vi "Drag-to-Dynamic.vi"(10 "Drag In":dbl, 11 "Waveform":waveform(dbl)) -> (3 "Dynamic Data Type":dynamicdata(waveform))   [LabVIEW 2025]
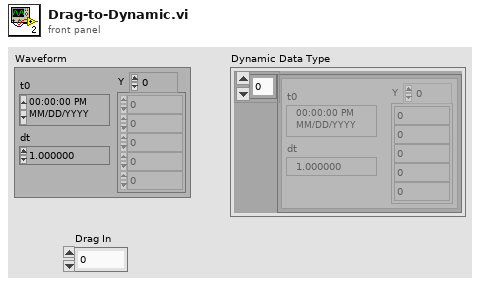
[diagram p1: front panel]
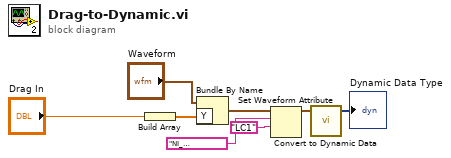
[diagram p0: block diagram]
diagram:
  n1 = Build Array("Drag In") -> (w8:dbl[])
  n2 = Bundle By Name(cluster="Waveform", "Y"=w8) -> (w2:waveform(dbl))
  n3 = Set Waveform Attribute(5:"LC1" ("name"), 6:"NI_ChannelName" ("name"), 7:w2) -> (3:w5:waveform(dbl))  [unwired: 1 in, 2 out]
  n4 = call "Convert to Dynamic Data"("Waveform"=w5) -> ("Dynamic Data Type"=→"Dynamic Data Type":dynamicdata)  [unwired: 3 in]
